vi "Target.vi"   [LabVIEW 2025]
uses:
  <vilib>/eio/utilities/niEioResolveVilibRelativePath.vi
  <vilib>/rvi/interface/RandomDataEmulation/niFpgaRandomDataHandleErrors.vi
  <vilib>/rvi/DataTransferAndStorage/Container/XNode/niFpgaContainer.xnode
  <vilib>/rvi/interface/RandomDataEmulation/nirviRandomDataFpgaReadWriteTemplate.vi
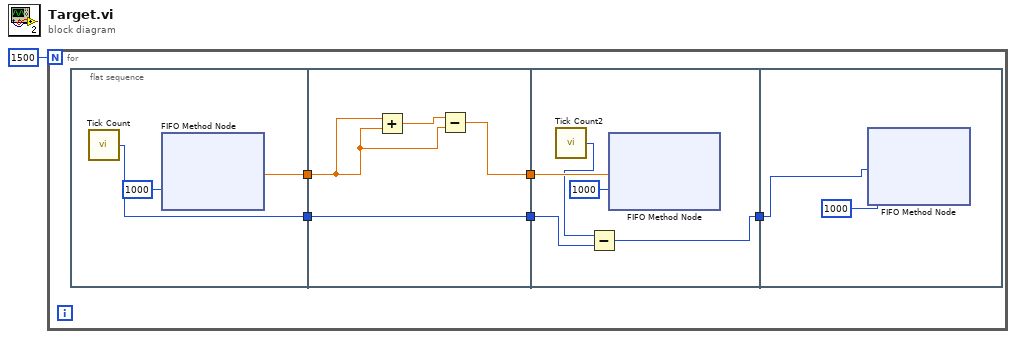
[diagram p0: block diagram]
diagram:
  n1 = for {
    N: 1500 -> [_]
    n2 = flat-sequence {
      tunnel: [w8] -> w5
      tunnel: [w7] -> w3
      tunnel: w5 -> [w11]
      tunnel: [w10] -> w4
      tunnel: w3 -> [w13]
      tunnel: [w13] -> w2
      tunnel: w4 -> [w18]
      tunnel: [w14] -> w6
      tunnel: w2 -> [w15]
      tunnel: w6 -> [w19]
      frame #0 {
        n3 = call "Tick Count"() -> ("Tick Count(Ticks)"=w7:u32)
        n4 = xnode ("FIFO Method Node")("Timeout"=1000) -> ("Element"=w8:sgl)  [unwired: 1 in, 2 out]
      }
      frame #1 {
        n5 = Add(x=w11, y=w11) -> (x+y=w12:sgl)
        n6 = Subtract(x=w12, y=w11) -> (x-y=w10:sgl)
      }
      frame #2 {
        n7 = call "Tick Count2"() -> ("Tick Count(Ticks)"=w16:u32)
        n8 = Subtract(x=w16, y=w15) -> (x-y=w14:u32)
        n9 = xnode ("FIFO Method Node")("Element"=w18, "Timeout"=1000) -> ()  [unwired: 1 in, 2 out]
      }
      frame #3 {
        n10 = xnode ("FIFO Method Node")("Element"=w19, "Timeout"=1000) -> ()  [unwired: 1 in, 2 out]
      }
    }
  }
